vi "Insight Example VI.vi"() -> ()   [LabVIEW 2012]
uses:
  <vilib>/Rock Robotics/SystemInterfaces/Typedef/FPGA_TypedefDigitalModule.ctl
panel:
  in  "Vision":dbl(slide) scale=-1.1..1.1
  in  "Scroll Timing":i32=1000
  in  "Distance":dbl format="%#_4f"
  in  "Arm Pot Value":dbl format="%#_5f"
  in  "Auto #":i32
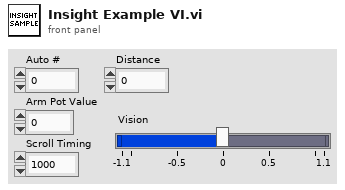
[diagram p1: front panel]
types:
  T1 = enum16{"FOUR_ZONES", "ONE_ZONE_TWO_LINES", "TWO_ZONES_ONE_LINE"}
  T2 = typedef "FPGA_TypedefDigitalModule.ctl" = enum16{"Digital Module 1", "Digital Module 2"}
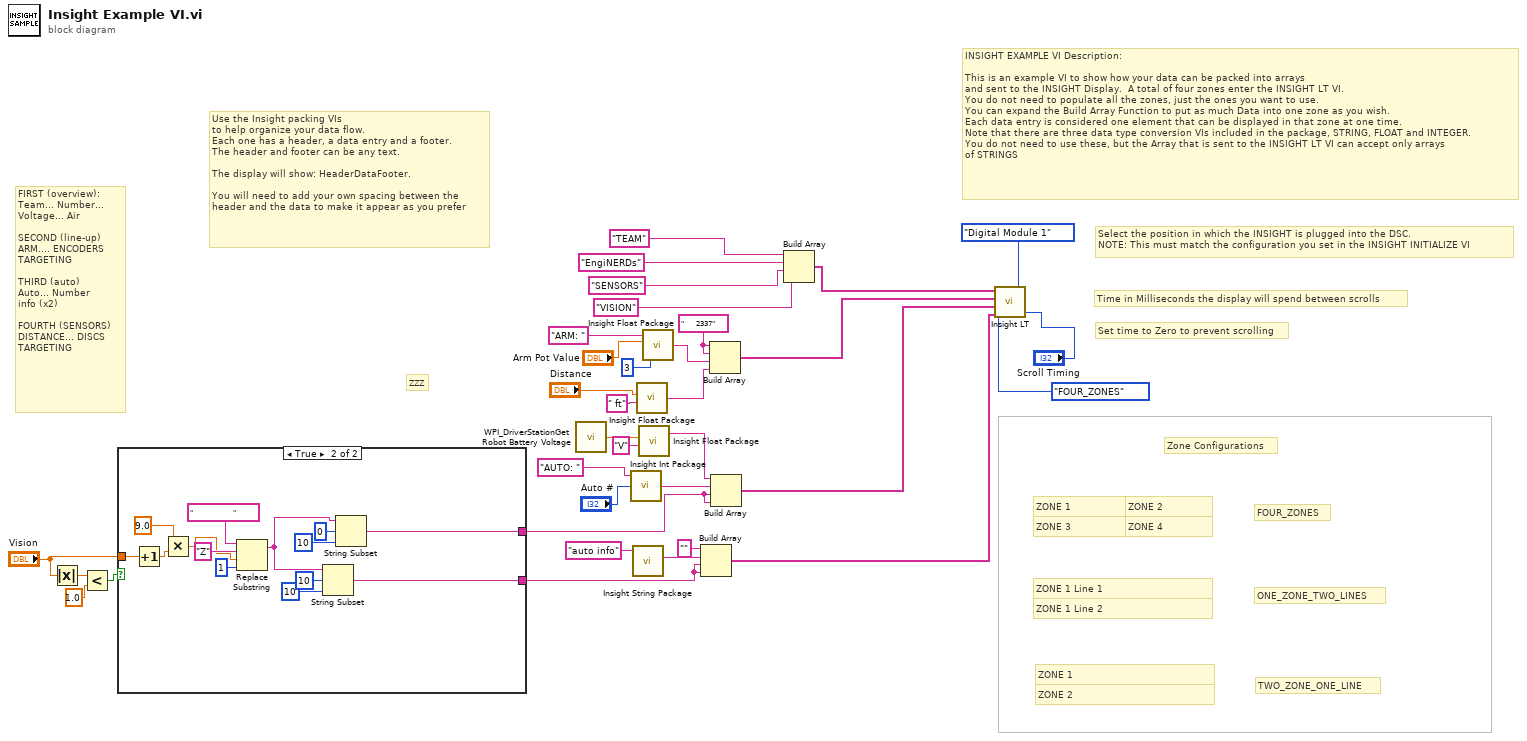
[diagram p0: block diagram]
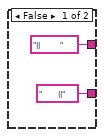
[diagram p2: hidden frame]
diagram:
  w23 = "      2337" ("element")
  # "ΖΖΖ"
  # "FIRST (overview): \nTeam... Number...\nVoltage... Air\n\nSECOND (line-up)\nARM.... ENCODERS\nTARGETING\n\nTHIRD (auto)\nAuto... Number\ninfo (x2)\n\nFOURTH (SENSORS)\nDISTANCE... DISCS\nTARGETING"
  # "Set time to Zero to prevent scrolling"
  # "Use the Insight packing VIs\nto help organize your data flow.\nEach one has a header, a data entry and a footer.\nThe header and footer can be any text.\n\nThe display will show: HeaderDataFooter.\n\nYou will need to add your own spacing between the \nheader and the data to make it appear as you prefer"
  # "TWO_ZONE_ONE_LINE"
  # "ONE_ZONE_TWO_LINES"
  # "FOUR_ZONES"
  # "Zone Configurations"
  # "ZONE 4"
  # "ZONE 2"
  # "ZONE 3"
  # "ZONE 1"
  # "ZONE 1 Line 2"
  # "ZONE 1 Line 1"
  # "ZONE 2"
  # "ZONE 1"
  # "Time in Milliseconds the display will spend between scrolls"
  # "Select the position in which the INSIGHT is plugged into the DSC.\nNOTE: This must match the configuration you set in the INSIGHT INITIALIZE VI"
  # "INSIGHT EXAMPLE VI Description:\n\nThis is an example VI to show how your data can be packed into arrays\nand sent to the INSIGHT Display.  A total of four zones enter the INSIGHT LT VI. \nYou do not need to populate all the zones, just the ones you want to use.\nYou can expand the Build Array Function to put as much Data into one zone as you wish.\nEach data entry is considered one element that can be displayed in that zone at one time.\nNote that there are three data type conversion VIs included in the package, STRING, FLOAT and INTEGER.\nYou do not need to use these, but the Array that is sent to the INSIGHT LT VI can accept only arrays\nof STRINGS"
  n1 = Absolute Value(x="Vision") -> (abs(x)=w5:dbl)
  n2 = Less?(x=w5, y=1.0) -> (x < y?=w3:bool)
  n3 = case shown="True" w3 {
    tunnel: "Vision" -> [_ w39]
    tunnel: ["||          " ("result string") w38] -> w1
    tunnel: ["        ||" ("result string") w37] -> w2
    frame False {
    }
    frame True {
      n4 = Increment(x=w39) -> (x+1=w49:dbl)
      n5 = Multiply(x=9.0, y=w49) -> (x*y=w40:dbl)
      n6 = Replace Substring(2:1 ("length (len. of substring)"), 3:w40, 4:"Ζ" ("substring (\"\")"), 5:"                    ") -> (1:w41:string)  [unwired: 1 out]
      n7 = String Subset(string=w41, offset (0)=10, length (rest)=10 ("length (rest)")) -> (substring=w37:string)
      n8 = String Subset(string=w41, offset (0)=0, length (rest)=10 ("length (rest)")) -> (substring=w38:string)
    }
  }
  n9 = call <vilib>:"WPI_DriverStationGet Robot Battery Voltage.vi"() -> ("robot battery voltage"=w31:dbl)  [unwired: 14 in, 1 out]
  n10 = call "Insight Int Package.vi"("Int32"="Auto #", "Header"="AUTO: " ("Footer")) -> ("resulting string"=w21:string)  [unwired: 1 in]
  n11 = call "Insight String Package.vi"("Header"="auto info" ("Footer")) -> ("resulting string"=w27:string)  [unwired: 2 in]
  n12 = call "Insight Float Package.vi"("Footer"=" ft", "Float"="Distance") -> ("resulting string"=w15:string)  [unwired: 2 in]
  n13 = call "Insight Float Package.vi"("Footer"="V", "Float"=w31) -> ("resulting string"=w9:string)  [unwired: 2 in]
  n14 = call "Insight Float Package.vi"("Decimal Places"=3, "Float"="Arm Pot Value", "Header"="ARM: ") -> ("resulting string"=w24:string)  [unwired: 1 in]
  n15 = Build Array("" ("element"), w27, w2, w2) -> (w10:string[])
  n16 = Build Array(w23, w23, w24, w15) -> (w20:string[])
  n17 = Build Array(w9, w21, w1, w1) -> (w25:string[])
  n18 = Build Array("TEAM" ("Header"), "EngiNERDs" ("Footer"), "SENSORS" ("Footer"), "VISION" ("element")) -> (w32:string[])
  n19 = call "Insight LT.vi"("Scroll Timing"="Scroll Timing", "ZONE \nCONFIGURATION"=T1."FOUR_ZONES" ("ZONE \nCONFIGURATION"), "Digital Module"=FPGA_TypedefDigitalModule."Digital Module 1", "Zone 4 Data"=w10, "Zone 3 Data"=w25, "Zone 2 Data"=w20, "Zone 1 Data"=w32) -> ()
